vi "log-fifo-uptoN.vi"(7 "N":i32, 8 "FIFO In":refnum<k21>="fpga-to-host2", 11 "input-data":fxp<+/-,25,6>[](array[numeric])=[0.0, 0.0, 0.0, 0.0, 0.0]) -> (3 "logging-timeout?":bool)   [LabVIEW 2017, in "FPGA-data-logging.lvlib"]
uses:
  FPGA-data-logging.lvlib
  <vilib>/rvi/DataTransferAndStorage/Container/Common/niFpgaContainerExecOnDevCompGetState.vi
  <vilib>/rvi/Emulation/niFpgaEmulationIsFPGAContextNoSignature.vi
  <vilib>/rvi/Emulation/niFpgaSctlEmulationGetInTimedLoop.vi
  <vilib>/rvi/errors/niFpgaSetErrorForExecOnDevCompSimple.vi
  <vilib>/rvi/eio/common/nirviEmuReportErrorAndStop.vi
  <vilib>/rvi/DataTransferAndStorage/Container/Common/niFpgaContainerGetUniqueNameForEmu.vi
  <vilib>/rvi/FIFO/Fifo_Resource/nirvififoEmulationSetSize.vi
  <vilib>/rvi/FIFO/Fifo_Resource/nirviFifoEmulationQueueMgr.vi
  <instcachedir>/0/nirviFifoEmulationQueueMgr_E5CAEC123FF24DC58D834DCA3CDAA9B5.lvgen/nirviFifoEmulationQueueMgr_E5CAEC123FF24DC58D834DCA3CDAA9B5_001.vi
  <vilib>/rvi/FIFO/Fifo_Resource/nirvififoEmulationDetermineInputValidOut.vi
  <vilib>/rvi/FIFO/Fifo_Resource/nirvififoEmulationCreateLock.vi
  <vilib>/rvi/Emulation/niFpgaProcessEmulError.vi
  <vilib>/rvi/FIFO/Fifo_Resource/nirvififoEmulationObtainLock.vi
  <vilib>/rvi/FIFO/Fifo_Resource/nirvififoEmulationReleaseLock.vi
  <vilib>/rvi/occurrence/nirviWaitOnOccurrenceBase.vi
  <vilib>/rvi/errors/nirviReportUnexpectedCaseInternalError.vi
  <vilib>/rvi/errors/nirviReportUnexpectedCaseInternalError (U32).vi
  <vilib>/Utility/error.llb/Clear Errors.vi
  <vilib>/rvi/interface/RandomDataEmulation/niFpgaRandomDataHandleErrors.vi
  <vilib>/rvi/DataTransferAndStorage/Container/XNode/niFpgaContainer.xnode
  <vilib>/rvi/FIFO/Fifo_Resource/niFpgaFifoEmulationRefIn.vi
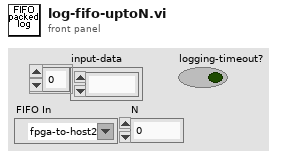
[diagram p1: front panel]
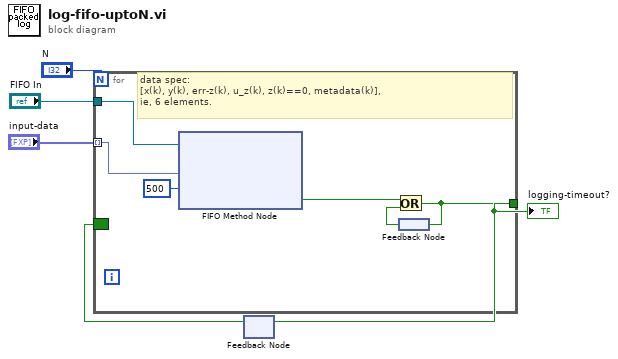
[diagram p0: block diagram]
diagram:
  n1 = feedback #1() -> (w3:bool)  [unwired: 1 in]
  n2 = for {
    N: "N" -> [_]
    tunnel: "input-data" -> [w11] mode=indexing
    tunnel: [w7] -> w5
    border: w3 -> [_]
    tunnel: "FIFO In" -> [w6]
    # "data spec:\n[x(k), y(k), err-z(k), u_z(k), z(k)==0, metadata(k)],\nie, 6 elements."
    n3 = xnode ("FIFO Method Node")("Element"=w11, "Timeout"=500, "FIFO In"=w6) -> ("Timed Out?"=w9:bool)  [unwired: 1 out]
    n4 = feedback #2() -> (w8:bool)
    n5 = Or(x=w9, y=w8) -> (x .or. y?=w7:bool)
    n6 = feedback-in #2(w7) -> ()
  }
  "logging-timeout?" <- w5
  n7 = feedback-in #1(w5) -> ()
